vi "Initialise.vi"(7 "Renderer":u32, 8 "error in (no error)":errorcluster) -> (0 "error out":errorcluster, 3 "Planet out":refnum<class "Planet.lvclass">)   [LabVIEW 2021, in "Planet.lvclass"]
uses:
  Planet.lvclass
  C:/dev/LabVIEW/LabMelee/Source/Application Specific/Element/Element.lvclass
  Planet Name.ctl
  Planet.lvclass/Planet.ctl
  <vilib>/numeric/Random Number (Range) U64.vi
  <vilib>/numeric/sub_Random U32.vi
  <vilib>/Utility/file.llb/Application Directory.vi
  Re-use Libraries/Vector 2D/Vector 2D.lvclass
  Element/Element.lvclass
  Resource Manager/Resource Manager.lvclass
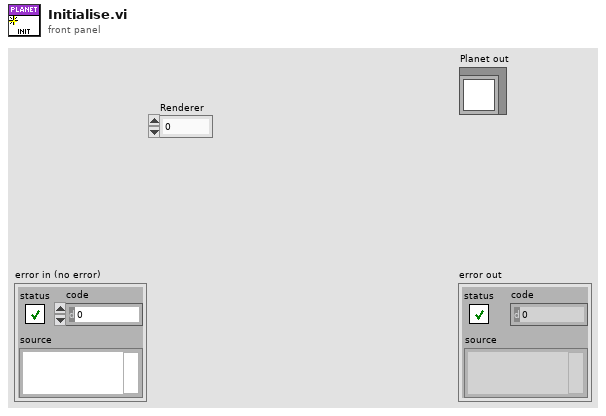
[diagram p1: front panel]
types:
  T1 = typedef "Planet.lvclass/Planet Name.ctl" = enum32{"acid", "alkali", "auric", "azure", "bluegas", "carbide", "chlorine", "chondrite", "cimmerian", "copper", "crimson", "cyangas", "cyanic", "dust", "earthmask", "emerald", "fluorescent", "green", "greengas", "greygas", "halide", "hydrocarbon", "infrared", "iodine", "lanthanide", "magma", "magnetic", "maroon", "metal", "noble", "oolite", "opalescent", "organic", "pellucid", "plutonic", "primordial", "purple", "purplegas", "quasidegenerate", "radioactive", "rainbow", "redgas", "redux", "ruby", "sapphire", "selenic", "shattered", "slaveshield", "superdense", "telluric", "treasure", "ultramarine", "urea", "vinylogous", "violetgas", "water", "xenolithic", "yellowgas"}
  T2 = typedef "Constants.ctl" = cluster{"Colours":cluster{"OK":u32, "Warning":u32, "Error":u32, "Red":u32, "Green":u32, "Blue":u32, "Yellow":u32}, "System":cluster{"Target Frames Second":dbl, "Windows Size":refnum<class "Vector 2D.lvclass">, "World Size":refnum<class "Vector 2D.lvclass">, "Battle Area Size":refnum<class "Vector 2D.lvclass">, "Sidebar Width":sgl, "SC2 Frame Rate [Seconds/Frame]":sgl, "Sidebar Player 2 Y Offset":sgl}, "Game":cluster{"Maximum Asteroids":i32, "Max Energy":i32, "Max Crew":i32, "Maximum Stars":i32}}
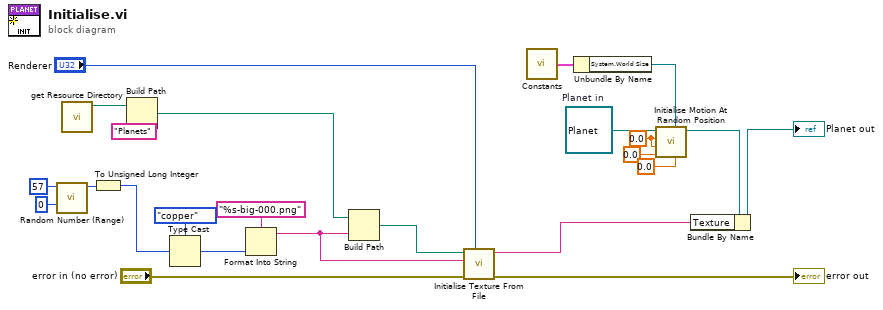
[diagram p0: block diagram]
diagram:
  w15 = sgl 0.0 ("Turn Rate [deg/s]")
  w21 = refnum<class "Planet.lvclass"> refnum  # Planet in
  n1 = call-poly <vilib>:"Random Number (Range).vi"("lower bound (0)"=u64 0, "upper bound (100)"=u64 57) -> ("number"=w2:u64)  [unwired: 9 in]
  n2 = call "get Resource Directory.vi"() -> ("Resource Directory"=w23:path)  [unwired: 11 in]
  n3 = To Unsigned Long Integer(number=w2) -> (unsigned 32bit integer=w1:u32)
  n4 = Build Path(base path=w23, name or relative path="Planets") -> (appended path=w16:path)
  n5 = Type Cast(type=Planet_Name."copper" ("Planet"), x=w1) -> (*(type *) &x=w9:T1)
  n6 = Format Into String(format string="%s-big-000.png", w9) -> (resulting string=w5:string)  [unwired: 2 in, 1 out]
  n7 = Build Path(base path=w16, name or relative path=w5) -> (appended path=w6:path)
  n8 = call "Initialise Texture From File.vi"("Renderer"="Renderer", "error in (no error)"="error in (no error)", "Name"=w5, "File"=w6) -> ("error out"=→"error out":errorcluster, "Name In Cache"=w3:string)  [unwired: 6 in]
  n9 = call "Constants.vi"() -> ("Constants"=w18:T2)
  n10 = Unbundle By Name(w18) -> ("System.World Size"=w17:refnum<class "Vector 2D.lvclass">)
  n11 = call "Initialise Motion At Random Position.vi"("Initial Velocity [m/s]"=sgl 0.0, "Field Size"=w17, "Maximum Velocity [m/s]"=sgl 0.0, "Acceleration [m/s/s]"=w15, "Turn Rate [deg/s]"=w15, "Element in"=w21) -> ("Element out"=w20:refnum<class "Planet.lvclass">)  [unwired: 5 in]
  n12 = Bundle By Name(cluster=w20, "Texture"=w3) -> (→"Planet out":refnum<class "Planet.lvclass">)
